vi "test_crest.vi"() -> ()   [LabVIEW 2014]
uses:
  common/crest/LabVIEW/LV14/libcommon-crest.lvlib
panel:
  out "JSON":string
  in  "cuname":string="BTF_SIM/DHSTB001"
  in  "!CHAOS WAN url":string="192.168.150.91:8081"
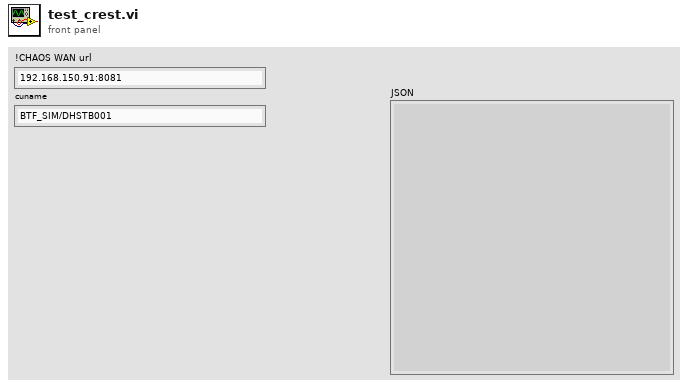
[diagram p1: front panel]
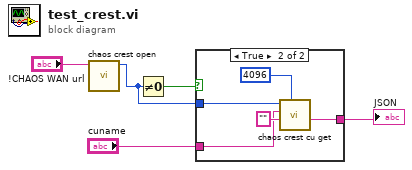
[diagram p0: block diagram]
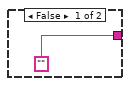
[diagram p2: hidden frame]
diagram:
  n1 = call "chaos crest open.vi"("chaoswanurl"="!CHAOS WAN url") -> ("function return"=w3:u32)  [unwired: 10 in]
  n2 = Not Equal To 0?(x=w3) -> (x != 0?=w4:bool)
  n3 = case shown="True" w4 {
    tunnel: w3 -> [_ w10]
    tunnel: "cuname" -> [_ w9]
    tunnel: ["" ("output out") w7] -> w1
    frame False {
    }
    frame True {
      n4 = call "chaos crest cu get.vi"("maxsize"=4096, "output"="", "cuname"=w9, "h"=w10) -> ("output out"=w7:string)  [unwired: 5 in, 2 out]
    }
  }
  "JSON" <- w1
